vi "Ejemplo.vi"() -> ()   [LabVIEW 2015, in "Arduino GIERM.lvlib"]
uses:
  <instrlib>/Arduino GIERM/Arduino GIERM.lvlib
panel:
  in  "VISA resource name":refnum<visa-resource-name>
  out "Disponible":bool
  in  "Baud Rate":u32=9600
  out "Valor":dbl
  in  "Stop Button":bool
  in  "Servo ON":bool
  in  "System ON":bool
  # "Torsion"
  # "USB Control"
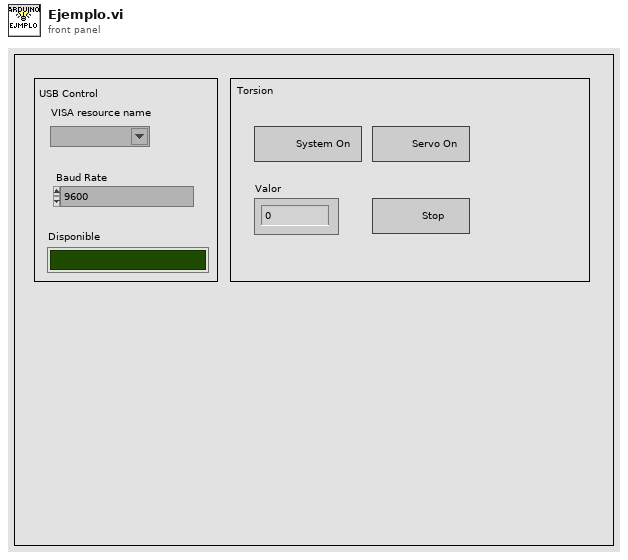
[diagram p1: front panel]
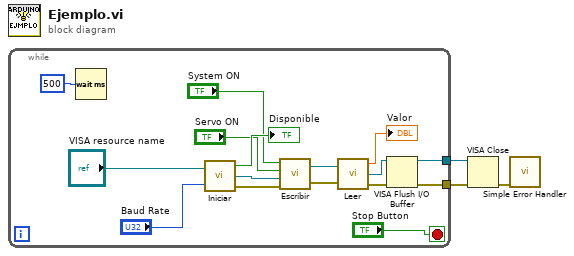
[diagram p0: block diagram]
diagram:
  n1 = while {
    tunnel: [w16] -> w2
    tunnel: [w17] -> w3
    stop <- "Stop Button" stop-if-true
    n2 = Wait (ms)(milliseconds to wait=u32 500 ("millisecond timer value")) -> ()  [unwired: 1 out]
    n3 = call <instrlib>:"Iniciar.vi"("VISA resource name"="VISA resource name", "baud rate (9600)"="Baud Rate") -> ("Disponible"=→"Disponible":bool, "VISA resource name 2"=w7:refnum<visa-resource-name>, "error out"=w6:errorcluster)
    n4 = call <instrlib>:"Escribir.vi"("error out"=w6, "VISA resource name out"=w7, "Servo ON"="Servo ON", "System ON"="System ON") -> ("error out 2"=w4:errorcluster, "VISA resource name out 2"=w5:refnum<visa-resource-name>)
    n5 = call <instrlib>:"Leer.vi"("VISA resource name out 2"=w5, "error out"=w4) -> ("Valor"=→"Valor":dbl, "VISA resource name out 3"=w11:refnum<visa-resource-name>, "error out 2"=w10:errorcluster)
    n6 = VISA Flush I/O Buffer(VISA resource name=w11, error in (no error)=w10) -> (VISA resource name out=w16:refnum<visa-resource-name>, error out=w17:errorcluster)  [unwired: 1 in]
  }
  n7 = VISA Close(VISA resource name=w2, error in (no error)=w3) -> (error out=w1:errorcluster)
  n8 = call <vilib>:"Simple Error Handler.vi"("error in (no error)"=w1) -> ()  [unwired: 4 in, 5 out]
